vi "hWaitonReady2014.vi"(4 "error in":errorcluster, 7 "FPGA VI Reference In":refnum<k20>) -> (0 "error out":errorcluster, 1 "Timeout":bool, 3 "FPGA VI Reference Out":refnum<k20>)   [LabVIEW 2014]
doc: "Wartet auf Ready-Signal. \nIst für Verwendung nach Selfcalibration der AD7730 gedacht"
uses:
  <vilib>/Utility/error.llb/Error Cluster From Error Code.vi
  <vilib>/rvi/errors/niLvFpgaAdjustHostInterfaceError.vi
  <vilib>/rvi/interface/nirviReadWriteControl/nirviReadWriteControl.xnode
  FPGA Bitfiles/W7XBolo2017_FPGATarget_FlorianDefault.lvbitx
  f_main_2014.vi
  NiFpgaLv.dll
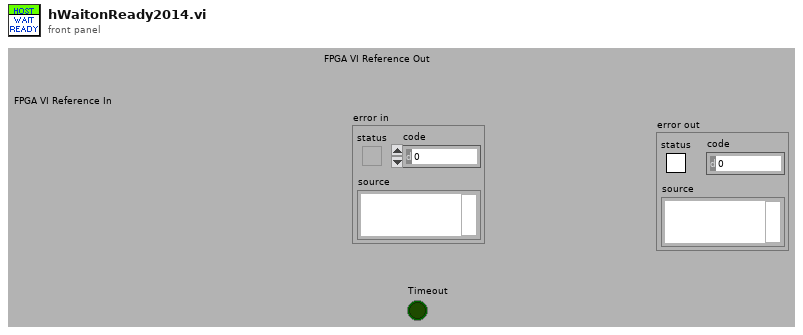
[diagram p1: front panel]
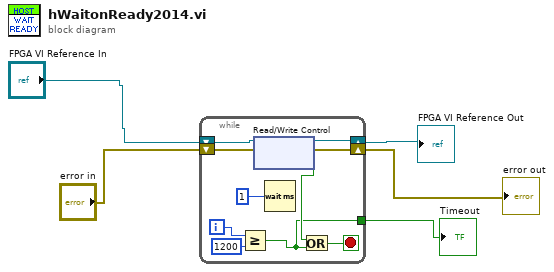
[diagram p0: block diagram]
diagram:
  n1 = while {
    tunnel: [w6] -> w3
    shift-right: [w13] -> w2
    shift-left: "FPGA VI Reference In" -> [w15]
    shift-right: [w12] -> w4
    shift-left: "error in" -> [w14]
    i -> [w10]
    stop <- w8 stop-if-true
    n2 = Greater Or Equal?(x=w10, y=1200) -> (x >= y?=w6:bool)
    n3 = xnode "Read/Write Control"("FPGA VI Reference In"=w15, "error in"=w14) -> ("FPGA VI Reference Out"=w13:refnum<k20>, "error out"=w12:errorcluster, "in Ready"=w7:bool)
    n4 = Wait (ms)(milliseconds to wait=1) -> ()  [unwired: 1 out]
    n5 = Or(x=w7, y=w6) -> (x .or. y?=w8:bool)
  }
  "error out" <- w4
  "Timeout" <- w3
  "FPGA VI Reference Out" <- w2
